vi "Dot or Comma.vi"() -> (0 "dot or comma":string)   [LabVIEW 2010, in "NI_Gmath.lvlib"]
uses:
  NI_Gmath.lvlib
panel:
  out "F-format string":string
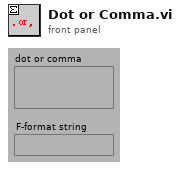
[diagram p1: front panel]
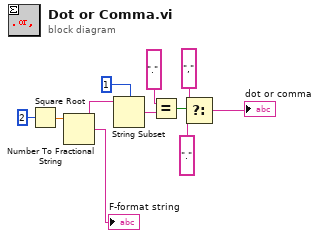
[diagram p0: block diagram]
diagram:
  w2 = 1
  n1 = Square Root(x=2) -> (sqrt(x)=w4:dbl)
  n2 = Number To Fractional String(number=w4) -> (F-format string=w1:string)  [unwired: 3 in]
  "F-format string" <- w1
  n3 = String Subset(string=w1, offset (0)=w2, length (rest)=w2) -> (substring=w5:string)
  n4 = Equal?(x=".", y=w5) -> (x = y?=w7:bool)
  n5 = Select(t=",", s=w7, f=".") -> (s? t:f=→"dot or comma":string)
